vi "Init.vi"(8 "error in":errorcluster, 11 "CANopen Master in":refnum<class "CANopen Master.lvclass">) -> (0 "error out":errorcluster, 3 "CANopen Master out":refnum<class "CANopen Master.lvclass">)   [LabVIEW 2024, in "CANopen Master.lvlib" / "CANopen Master.lvclass"]
uses:
  CANopen Master.lvclass
  CANopen Master.lvclass/CANopen Master.ctl
  SDO Manager/SDO Manager.lvclass
  Example/Network Management/Network Mangement.lvclass
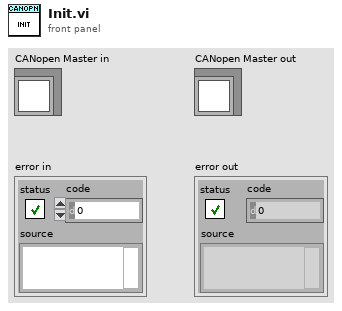
[diagram p1: front panel]
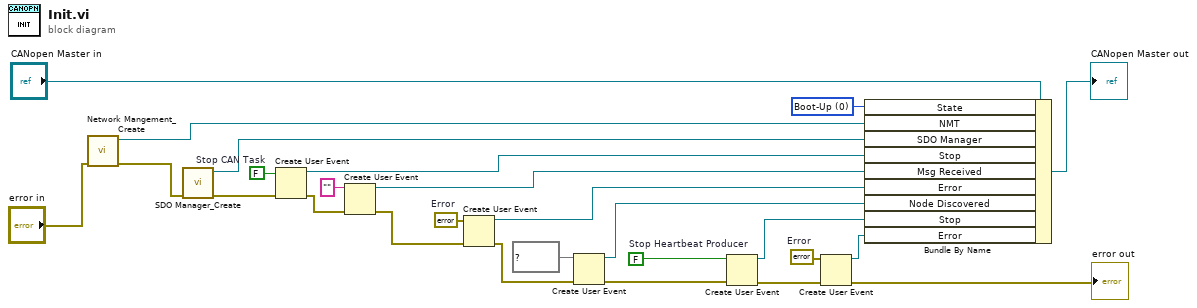
[diagram p0: block diagram]
diagram:
  w2 = FALSE  # Stop Heartbeat Producer
  w3 = errorcluster {"status"=FALSE, "code"=0, "source"=""}  # Error
  w8 = u16 0 items=["Boot-Up"=0, "Stopped"=4, "Operational"=5, "Pre-Operational"=127] ("State")
  w13 = errorcluster {"status"=FALSE, "code"=0, "source"=""}  # Error
  w20 = FALSE  # Stop CAN Task
  n1 = call "Network Mangement_Create.vi"("Error In"="error in") -> ("Error Out"=w9:errorcluster, "reference out"=w24:refnum<class "Network Mangement.lvclass">)  [unwired: 9 in]
  n2 = call "SDO Manager_Create.vi"("Error In"=w9) -> ("Error Out"=w21:errorcluster, "reference out"=w25:refnum<class "SDO Manager.lvclass">)  [unwired: 9 in]
  n3 = Create User Event(user event datatype=w20, error in=w21) -> (user event=w19:refnum<user-event>, error out=w17:errorcluster)
  n4 = Create User Event(user event datatype="" ("Message Received"), error in=w17) -> (user event=w15:refnum<user-event>, error out=w16:errorcluster)
  n5 = Create User Event(user event datatype=w13, error in=w16) -> (user event=w10:refnum<user-event>, error out=w14:errorcluster)
  n6 = Create User Event(user event datatype=map{u8, u8} {} ("Nodes"), error in=w14) -> (user event=w12:refnum<user-event>, error out=w7:errorcluster)
  n7 = Create User Event(user event datatype=w2, error in=w7) -> (user event=w6:refnum<user-event>, error out=w5:errorcluster)
  n8 = Create User Event(user event datatype=w3, error in=w5) -> (user event=w4:refnum<user-event>, error out=→"error out":errorcluster)
  n9 = Bundle By Name(cluster="CANopen Master in", "State"=w8, "NMT"=w24, "SDO Manager"=w25, "Stop"=w19, "Msg Received"=w15, "Error"=w10, "Node Discovered"=w12, "Stop"=w6, "Error"=w4) -> (→"CANopen Master out":refnum<class "CANopen Master.lvclass">)
